vi "DAQ Finite Read Servo Errors.vi"(5 "samples per channel":i32=1000, 7 "rate":dbl=1000.0 caption="Samples per Second" format="%0.2f", 8 "error in":errorcluster, 10 "task/channels in":refnum<k21>, 11 "Action":T1) -> (0 "error out":errorcluster, 2 "Average":dbl[](array[numeric]))   [LabVIEW 2009]
uses:
  DAQ Read Actions.ctl
  <vilib>/DAQmx/configure/timing.llb/DAQmx Timing (Sample Clock).vi
  <vilib>/DAQmx/read.llb/DAQmx Read (Analog 2D DBL NChan NSamp).vi
panel:
  out "Data":dbl[][](array[numeric]) format="%0.2f"
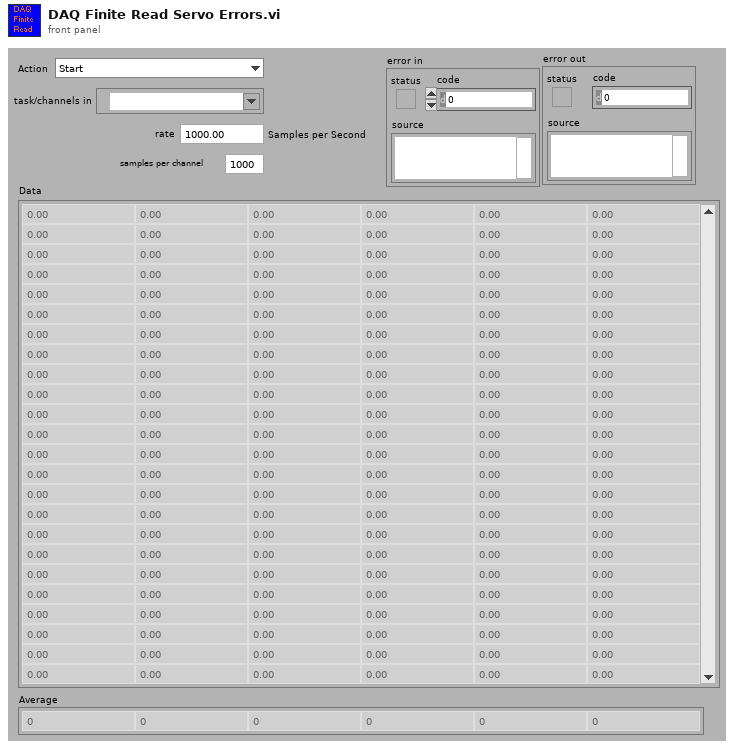
[diagram p1: front panel]
types:
  T1 = typedef "DAQ Read Actions.ctl" = enum16{"Start", "Read", "Stop"}
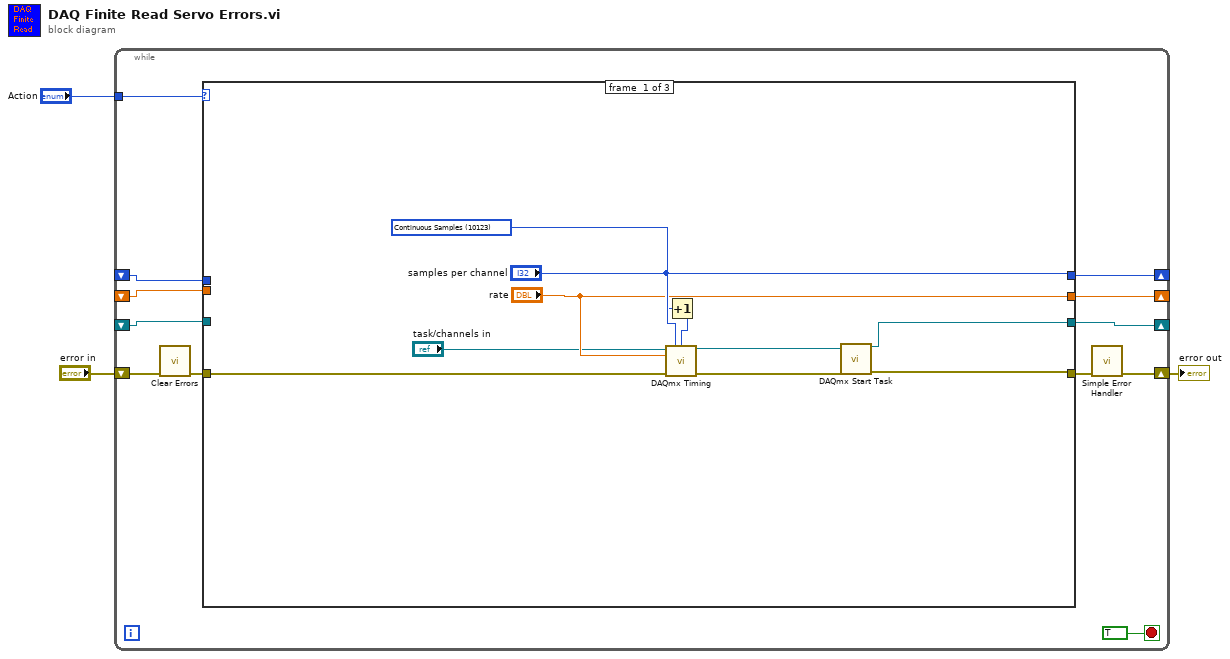
[diagram p0: block diagram]
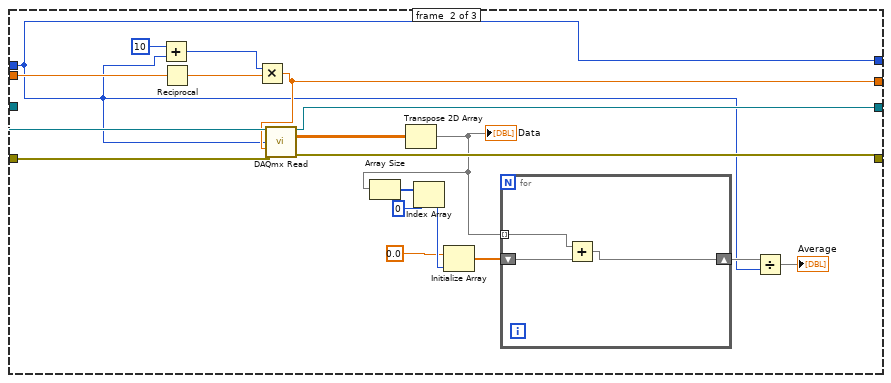
[diagram p2: hidden frame]
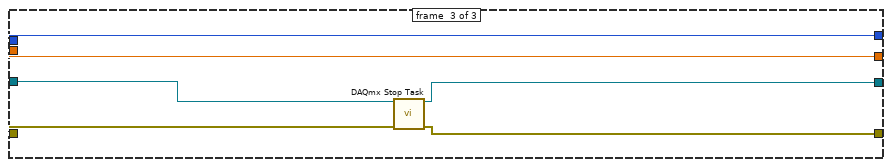
[diagram p3: hidden frame]
diagram:
  n1 = while {
    tunnel: "Action" -> [w14]
    shift-right: [w5] -> w2
    shift-left: "error in" -> [w12]
    shift-right: [w11] -> _
    shift-left: _ -> [w10]
    shift-right: [w8] -> _
    shift-left: _ -> [w6]
    shift-right: [w9] -> _
    shift-left: _ -> [w7]
    stop <- TRUE stop-if-true
    n2 = call <vilib>:"Clear Errors.vi"("error in (no error)"=w12) -> ("error out"=w4:errorcluster)  [unwired: 6 out]
    n3 = case shown="\"Read\"" w14 {
      tunnel: [w17 w43 w50] -> w13
      tunnel: w4 -> [w21 w39 w52]
      tunnel: [w18 w44 w51] -> w11
      tunnel: w10 -> [_ w38 w53]
      tunnel: ["samples per channel" w26 w48] -> w9
      tunnel: ["rate" w28 w49] -> w8
      tunnel: w7 -> [_ w26 w48]
      tunnel: w6 -> [_ w42 w49]
      frame #0 {
        w25 = 10123 items=["Finite Samples"=10178, "Continuous Samples"=10123, "Hardware Timed Single Point"=12522] ("sample mode")
        n4 = Increment(x="samples per channel") -> (x+1=w16:i32)
        n5 = call-poly <vilib>:"DAQmx Timing.vi"("task/channels in"="task/channels in", "sample mode"=w25, "samples per channel"=w16, "rate"="rate", "error in"=w21) -> ("task out"=w19:refnum<k21>, "error out"=w20:errorcluster)  [unwired: 2 in, 7 out]
        n6 = call <vilib>:"DAQmx Start Task.vi"("task/channels in"=w19, "error in"=w20) -> ("task out"=w18:refnum<k21>, "error out"=w17:errorcluster)  [unwired: 12 out]
      }
      frame #1 {
        n7 = Add(x=10, y=w26) -> (x+y=w37:i32)
        n8 = Reciprocal(x=w42) -> (1/x=w27:dbl)
        n9 = Multiply(x=w37, y=w27) -> (x*y=w28:dbl)
        n10 = call-poly <vilib>:"DAQmx Read.vi"("task/channels in"=w38, "number of samples per channel"=w26, "timeout"=w28, "error in"=w39) -> ("task out"=w44:refnum<k21>, "data"=w40:dbl[][], "error out"=w43:errorcluster)  [unwired: 9 out]
        n11 = Transpose 2D Array(2D array=w40) -> (transposed array=w34:dbl[][])
        "Data" <- w34
        n12 = Array Size(array=w34) -> (size(s)=w33:i32[])
        n13 = Index Array(array=w33, index=0) -> (element=w30:i32)
        n14 = Initialize Array(0.0 ("element"), w30) -> (w31:dbl[])
        n15 = for {
          shift-right: [w46] -> w36
          shift-left: w31 -> [w45]
          tunnel: w34 -> [w47] mode=indexing
          n16 = Add(x=w47, y=w45) -> (x+y=w46:dbl[])
        }
        n17 = Divide(x=w36, y=w26) -> (x/y=→"Average":dbl[])
      }
      frame #2 {
        n18 = call <vilib>:"DAQmx Stop Task.vi"("task/channels in"=w53, "error in"=w52) -> ("task out"=w51:refnum<k21>, "error out"=w50:errorcluster)  [unwired: 12 out]
      }
    }
    n19 = call <vilib>:"Simple Error Handler.vi"("error in (no error)"=w13) -> ("error out"=w5:errorcluster)  [unwired: 1 in, 7 out]
  }
  "error out" <- w2
